vi "Video File Close.vi"(8 "error in (no error)":errorcluster, 11 "Realsense Cam File Wrapper in":refnum<class "Realsense Cam File Wrapper.lvclass">) -> (0 "error out":errorcluster, 3 "Realsense Cam File Wrapper out":refnum<class "Realsense Cam File Wrapper.lvclass">)   [LabVIEW 2018, in "Realsense Cam File Wrapper.lvclass"]
uses:
  Realsense Cam File Wrapper.lvclass
  Realsense Cam File Wrapper.lvclass/Realsense Cam File Wrapper.ctl
  Realsense Cam/Realsense Cam.lvclass
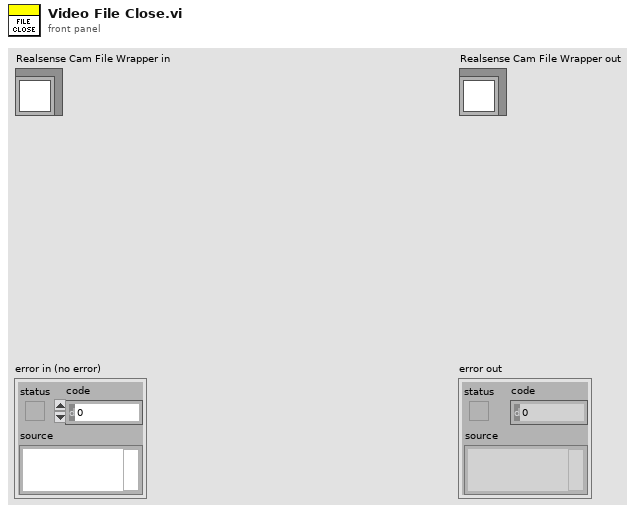
[diagram p1: front panel]
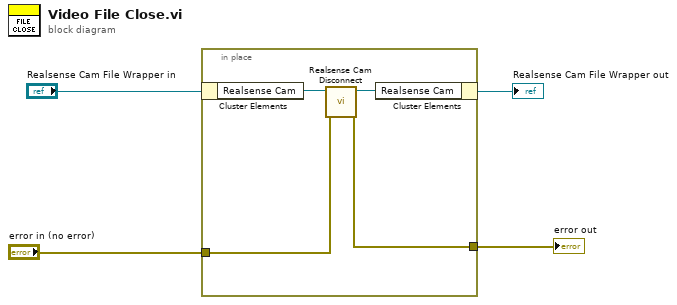
[diagram p0: block diagram]
diagram:
  n1 = in-place {
    in-place-border: "error in (no error)" -> [w6]
    in-place-border: [w5] -> w1
    n2 = in-place-cluster #1("Realsense Cam File Wrapper in") -> ("Realsense Cam"=w8:refnum<class "Realsense Cam.lvclass">)
    n3 = call-dynamic "Realsense Cam Disconnect.vi"("error in (no error)"=w6, "Realsense Cam in"=w8) -> ("error out"=w5:errorcluster, "Realsense Cam out"=w7:refnum<class "Realsense Cam.lvclass">)  [unwired: 7 in, 1 out]
    n4 = in-place-cluster #1("Realsense Cam"=w7) -> (→"Realsense Cam File Wrapper out":refnum<class "Realsense Cam File Wrapper.lvclass">)
  }
  "error out" <- w1
